vi "Keithley 2400 Voltage Read.vi"(8 "error in (no error)":errorcluster, 11 "VISA Refnum in":refnum<visa-resource-name>) -> (0 "error out":errorcluster, 3 "Voltage Reading":dbl)   [LabVIEW 2019]
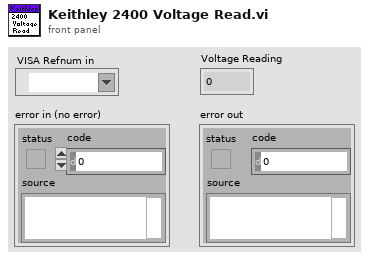
[diagram p1: front panel]
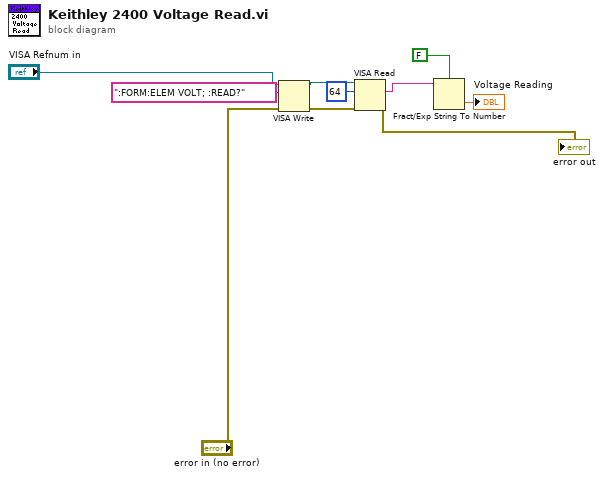
[diagram p0: block diagram]
diagram:
  n1 = VISA Write(VISA resource name="VISA Refnum in", write buffer=":FORM:ELEM VOLT; :READ?", error in (no error)="error in (no error)") -> (VISA resource name out=w5:refnum<visa-resource-name>, error out=w4:errorcluster)  [unwired: 1 out]
  n2 = VISA Read(VISA resource name=w5, byte count=u32 64, error in (no error)=w4) -> (read buffer=w7:string, error out=→"error out":errorcluster)  [unwired: 2 out]
  n3 = Fract/Exp String To Number(use system decimal point (T)=FALSE, string=w7) -> (number=→"Voltage Reading":dbl)  [unwired: 2 in, 1 out]
